vi "ProjectOpenReferences.vi"(0 "Project File Path":path, 5 "Gateway IP Address (\"\": localhost)":string, 11 "error in (no error)":errorcluster, 12 "Username":string, 13 "Password":string) -> (4 "Project File Path out":path, 6 "Gateway IP Address out":string, 15 "error out":errorcluster)   [LabVIEW 2015, in "ni-veristand-steps-runtime-lib.lvlib"]
uses:
  ni-veristand-steps-runtime-lib.lvlib
  controls/VeriStand dotNet References.ctl
  NationalInstruments.VeriStand.ClientAPI
  <vilib>/NI Veristand/Execution/Workspace/NI_VS Workspace ExecutionAPI.lvlib
  <vilib>/NI Veristand/Execution/ChannelFaultManager/NI_VS ChannelFault ExecutionAPI.lvlib
  <vilib>/NI Veristand/Execution/ModelManager/NI_VS ModelManager ExecutionAPI.lvlib
  <vilib>/NI Veristand/Execution/Project/NI_VS Project ExecutionAPI.lvlib
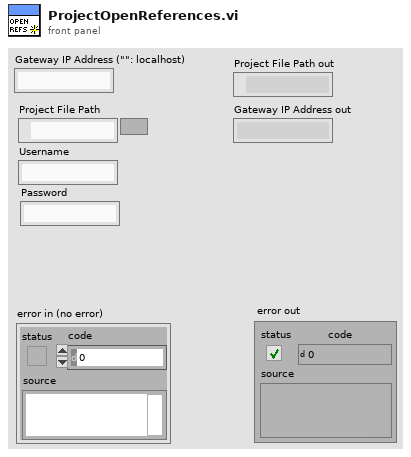
[diagram p1: front panel]
types:
  T1 = typedef "ni-veristand-steps-runtime-lib.lvlib/VeriStand dotNet References.ctl" = cluster{"Project Ref":refnum<k24>, "Workspace Manager Ref":refnum<k24>, "Model Manager Ref":refnum<k24>, "Channel Fault Manager Ref":refnum<k24>}
  T2 = typedef "NI_VS Workspace ExecutionAPI.lvlib/WorkspaceAPI.ctl" = refnum<k24>
  T3 = typedef "NI_VS ModelManager ExecutionAPI.lvlib/ModelManagerAPI.ctl" = refnum<k24>
  T4 = typedef "NI_VS ChannelFault ExecutionAPI.lvlib/ChannelFaultAPI.ctl" = refnum<k24>
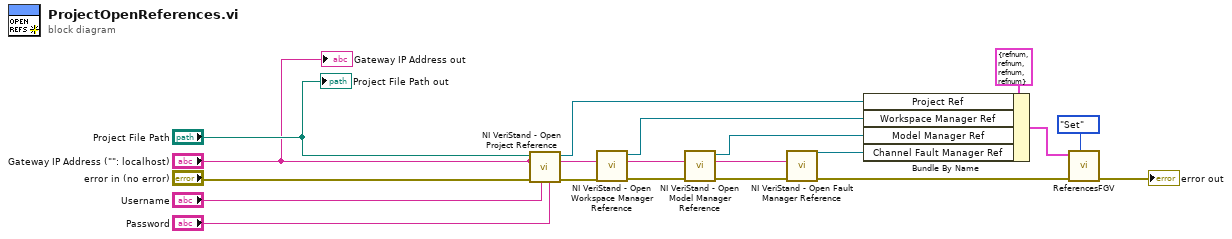
[diagram p0: block diagram]
diagram:
  n1 = call <vilib>:"NI VeriStand - Open Project Reference.vi"("Password"="Password", "Username"="Username", "error in (no error)"="error in (no error)", "Gateway IP Address (\"\": localhost)"="Gateway IP Address (\"\": localhost)", "Project File Path"="Project File Path") -> ("error out"=w2:errorcluster, "Project Ref"=w1:refnum<k24>)  [unwired: 5 in]
  n2 = call <vilib>:"NI VeriStand - Open Workspace Manager Reference.vi"("error in (no error)"=w2, "Gateway IP Address (\"\": localhost)"="Gateway IP Address (\"\": localhost)") -> ("error out"=w17:errorcluster, "WorkspaceManager"=w10:T2)  [unwired: 8 in]
  n3 = call <vilib>:"NI VeriStand - Open Model Manager Reference.vi"("error in (no error)"=w17, "Gateway IP Address (\"\": localhost)"="Gateway IP Address (\"\": localhost)") -> ("error out"=w16:errorcluster, "ModelManager"=w9:T3)  [unwired: 8 in]
  n4 = call <vilib>:"NI VeriStand - Open Fault Manager Reference.vi"("error in (no error)"=w16, "Gateway IP Address (\"\": localhost)"="Gateway IP Address (\"\": localhost)") -> ("error out"=w6:errorcluster, "ChannelFault"=w7:T4)  [unwired: 8 in]
  n5 = Bundle By Name(cluster=T1 {"Project Ref"=refnum, "Workspace Manager Ref"=refnum, "Model Manager Ref"=refnum, "Channel Fault Manager Ref"=refnum} ("VeriStand dotNET Refs"), "Project Ref"=w1, "Workspace Manager Ref"=w10, "Model Manager Ref"=w9, "Channel Fault Manager Ref"=w7) -> (w5:T1)
  n6 = call "ReferencesFGV.vi"("Get/Set"=enum16{"Get", "Set"}."Set", "error in (no error)"=w6, "VeriStand dotNET Refs"=w5) -> ("error out"=→"error out":errorcluster)  [unwired: 7 in, 1 out]
  "Project File Path out" <- "Project File Path"
  "Gateway IP Address out" <- "Gateway IP Address (\"\": localhost)"
